vi "Read Device Identification.vi"(8 "error in (no error)":errorcluster, 9 "object ID":u8, 10 "device ID category":T1(ring), 11 "Modbus slave in":refnum<class "Modbus Slave.lvclass">) -> (0 "error out":errorcluster, 2 "objects":cluster{"object ID":u8, "value":string}[](array[cluster]) {"object ID" format="%x"}, 3 "Modbus slave out":refnum<class "Modbus Slave.lvclass">)   [LabVIEW 2017, in "Modbus Slave.lvclass"]
doc: "Returns the device identification of a Modbus slave. Device identification consists of data elements called objects. Each object has an identification number and stores Modbus slave information."
uses:
  <vilib>/Modbus/slave/Modbus Slave.lvclass
  <vilib>/Modbus/slave/Modbus Slave.lvclass/Modbus Slave.ctl
  <vilib>/Modbus/subvis/Data and Functions/Device Data Model/Device Data Model.lvclass
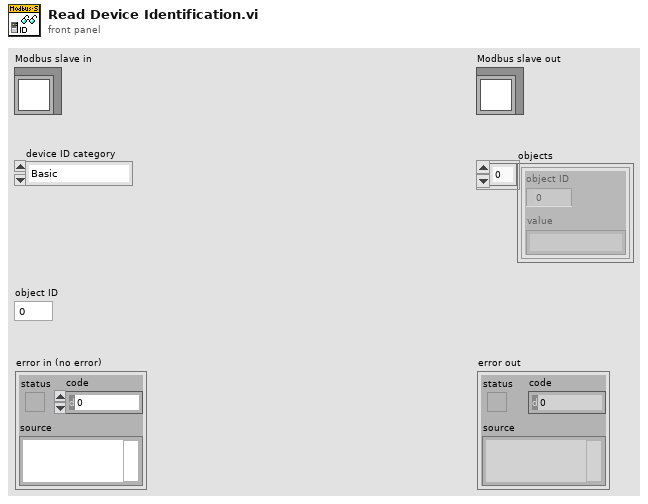
[diagram p1: front panel]
types:
  T1 = enum8{"Basic", "Regular", "Extended", "Specific"}
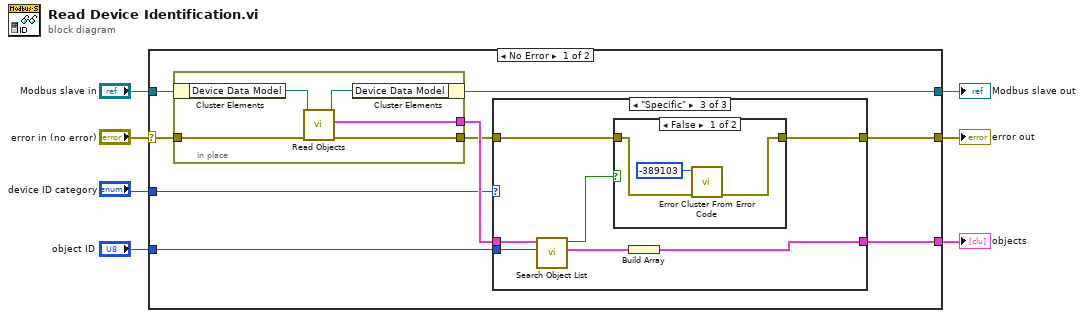
[diagram p0: block diagram]
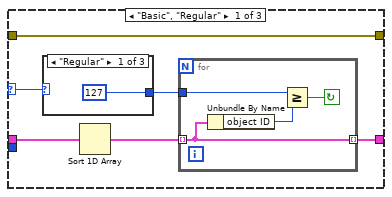
[diagram p2: hidden frame]
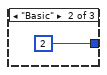
[diagram p3: hidden frame]
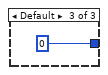
[diagram p4: hidden frame]
diagram:
  n1 = case shown="No Error" "error in (no error)" {
    selector: "error in (no error)" -> [w8 w48]
    tunnel: [w16 w49] -> w7
    tunnel: "Modbus slave in" -> [w15 w49]
    tunnel: "device ID category" -> [w13 _]
    tunnel: "object ID" -> [w12 _]
    tunnel: [w11 _] -> w4
    tunnel: [w10 w48] -> w3
    frame No Error {
      n2 = in-place {
        in-place-border: [w47] -> w14
        in-place-border: [w46] -> w9
        in-place-border: w8 -> [w45]
        n3 = in-place-cluster #1(w15) -> ("Device Data Model"=w44:refnum<class "Device Data Model.lvclass">)
        n4 = call-dynamic "Read Objects.vi"("error in (no error)"=w45, "device data model in"=w44) -> ("error out"=w46:errorcluster, "objects"=w47:cluster{"object ID":u8, "value":string}[], "device data model out"=w43:refnum<class "Device Data Model.lvclass">)  [unwired: 7 in]
        n5 = in-place-cluster #1("Device Data Model"=w43) -> (w16:refnum<class "Modbus Slave.lvclass">)
      }
      n6 = case shown="\"Specific\"" w13 {
        selector: w13 -> [w19 _ _]
        tunnel: w14 -> [w20 w30 w38]
        tunnel: w9 -> [w22 w31 w33]
        tunnel: w12 -> [_ _ w37]
        tunnel: [w21 w30 w34] -> w11
        tunnel: [w22 w31 w32] -> w10
        frame "Basic", "Regular" {
          n7 = case shown="\"Regular\"" w19 {
            tunnel: [u8 127 ("y") u8 2 ("y") u8 0 ("y")] -> w18
            frame "Regular" {
            }
            frame "Basic" {
            }
            frame Default {
            }
          }
          n8 = Sort 1D Array(array=w20) -> (sorted array=w17:cluster{"object ID":u8, "value":string}[])
          n9 = for {
            tunnel: w17 -> [w29] mode=indexing
            tunnel: [w29] -> w21 mode=indexing
            tunnel: w18 -> [w27]
            stop <- w28 continue-if-true
            n10 = Unbundle By Name(w29) -> ("object ID"=w26:u8)
            n11 = Greater Or Equal?(x=w27, y=w26) -> (x >= y?=w28:bool)
          }
        }
        frame "Extended" {
        }
        frame "Specific" {
          n12 = call <vilib>:"Search Object List.vi"("object ID"=w37, "objects"=w38) -> ("object"=w35:cluster{"object ID":u8, "value":string}, "found?"=w36:bool)  [unwired: 7 in, 1 out]
          n13 = case shown="False" w36 {
            tunnel: w33 -> [w40 w42]
            tunnel: [w41 w42] -> w32
            frame False {
              n14 = call <vilib>:"Error Cluster From Error Code.vi"("error in (no error)"=w40, "error code (0)"=-389103) -> ("error out"=w41:errorcluster)  [unwired: 7 in]
            }
            frame True {
            }
          }
          n15 = Build Array(w35) -> (w34:cluster{"object ID":u8, "value":string}[])
        }
      }
    }
    frame Error {
    }
  }
  "error out" <- w3
  "Modbus slave out" <- w7
  "objects" <- w4
